vi "Wave1D_Cal Uk.vi"(10 "time step":i32, 11 "Wave1D Data In":T1 {"BC"."End X"."type" items=["Dirichlet", "Neumann"]; "BC"."Start X"."type" items=["Dirichlet", "Neumann"]}) -> (3 "Wave1D Data Out":T1 {"BC"."End X"."type" items=["Dirichlet", "Neumann"]; "BC"."Start X"."type" items=["Dirichlet", "Neumann"]})   [LabVIEW 2017, in "NI_PDE.lvlib"]
uses:
  <vilib>/gmath/NI_PDE.lvlib
  <vilib>/gmath/pde.llb/Wave1D/Wave1D_Data.ctl
  <vilib>/gmath/pde.llb/Common/PDE_BC Type.ctl
  <vilib>/Analysis/Matrix/Datatypes/RealMatrix.ctl
  <vilib>/Analysis/Matrix/NI_Matrix.lvlib
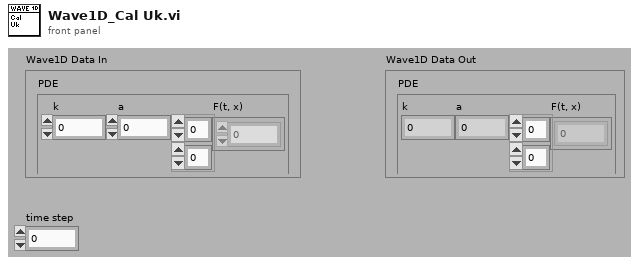
[diagram p1: front panel]
types:
  T1 = typedef "NI_PDE.lvlib/Wave1D_Data.ctl" = cluster{"PDE":cluster{"k":dbl, "a":dbl, "F(t, x)":dbl[][]}, "Domain":cluster{"t":cluster{"initial t":dbl, "final t":dbl, "# of t-points":i32}, "x":cluster{"start x":dbl, "end x":dbl, "# of x-points":i32}, "delta":cluster{"delta t":dbl, "delta x":dbl}}, "BC":cluster{"Start X":cluster{"type":T2, "Value":dbl[]}, "End X":cluster{"type":T2, "Value":dbl[]}}, "IC":cluster{"Value":dbl[], "Derivative":dbl[]}, "A":cluster{"Sub Diag":dbl[], "Diag":dbl[], "Super Diag":dbl[], "A":T3}, "LU of A":cluster{"L":dbl[], "U":cluster{"Diag":dbl[], "Super Diag":dbl[], "2nd Super Diag":dbl[]}, "Pivot":i32[]}, "State":cluster{"U":dbl[], "AU":dbl[], "Old AU":dbl[], "start index":i32, "length":i32}}
  T2 = typedef "NI_PDE.lvlib/PDE_BC Type.ctl" = i32
  T3 = typedef "NI_Matrix.lvlib/RealMatrix.ctl" = dbl[][]
  T4 = cluster{"Sub Diag":dbl[], "Diag":dbl[], "Super Diag":dbl[], "A":T3}
  T5 = cluster{"L":dbl[], "U":cluster{"Diag":dbl[], "Super Diag":dbl[], "2nd Super Diag":dbl[]}, "Pivot":i32[]}
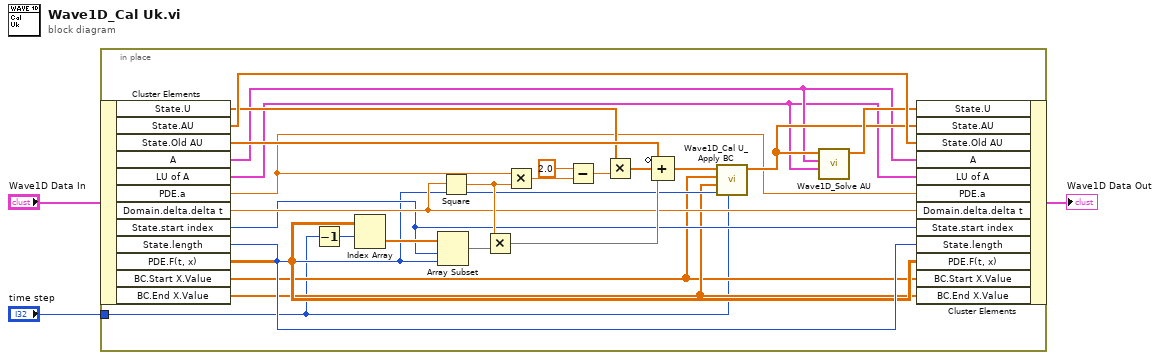
[diagram p0: block diagram]
diagram:
  n1 = in-place {
    in-place-border: "time step" -> [w4]
    n2 = in-place-cluster #1("Wave1D Data In") -> ("State.U"=w14:dbl[], "State.AU"=w18:dbl[], "State.Old AU"=w15:dbl[], "A"=w13:T4, "LU of A"=w12:T5, "PDE.a"=w11:dbl, "Domain.delta.delta t"=w10:dbl, "State.start index"=w9:i32, "State.length"=w8:i32, "PDE.F(t, x)"=w7:dbl[][], "BC.Start X.Value"=w5:dbl[], "BC.End X.Value"=w6:dbl[])
    n3 = Decrement(x=w4) -> (x-1=w19:i32)
    n4 = Index Array(array=w7, index (row)=w19) -> (element=w25:dbl[])  [unwired: 1 in]
    n5 = Array Subset(array=w25, index=w9, length=w8) -> (w24:dbl[])
    n6 = Square(x=w10) -> (x^2=w21:dbl)
    n7 = Multiply(x=w21, y=w24) -> (x*y=w22:dbl[])
    n8 = Multiply(x=w11, y=w21) -> (x*y=w28:dbl)
    n9 = Subtract(x=2.0, y=w28) -> (x-y=w26:dbl)
    n10 = Multiply(x=w14, y=w26) -> (x*y=w23:dbl[])
    n11 = Compound Arithmetic op=ADD(invert w15, w23, w22) -> (w20:dbl[])
    n12 = call <vilib>:"Wave1D_Cal U_Apply BC.vi"("time step"=w4, "length"=w8, "End X Value"=w6, "Start X Value"=w5, "U In"=w20) -> ("U Out"=w16:dbl[])  [unwired: 6 out]
    n13 = call <vilib>:"Wave1D_Solve AU.vi"("LU of A"=w12, "A"=w13, "U"=w16) -> ("A\\U"=w17:dbl[])  [unwired: 8 out]
    n14 = in-place-cluster #1("State.U"=w17, "State.AU"=w16, "State.Old AU"=w18, "A"=w13, "LU of A"=w12, "PDE.a"=w11, "Domain.delta.delta t"=w10, "State.start index"=w9, "State.length"=w8, "PDE.F(t, x)"=w7, "BC.Start X.Value"=w5, "BC.End X.Value"=w6) -> (→"Wave1D Data Out":T1)
  }
